vi "Config Write Interface.vi"(8 "error in (no error)":errorcluster, 10 "Device Ref in":T1 format="%.0x", 11 "Refnum in":T2) -> (0 "error out":errorcluster, 2 "Device Ref out":T1 format="%.0x", 3 "Refnum out":T2)   [LabVIEW 2019, in "Modbus Master System Explorer.lvlib"]
uses:
  Modbus Master System Explorer.lvlib
  <vilib>/Utility/config.llb/Config Data RefNum.ctl
  <vilib>/NI VeriStand/Custom Device API/Custom Device Item Ref.ctl
  <vilib>/Utility/config.llb/NI_LVConfig.lvlib
  <vilib>/NI VeriStand/Custom Device API/Custom Device API.lvlib
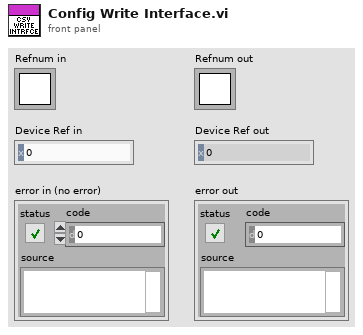
[diagram p1: front panel]
types:
  T1 = typedef "Custom Device API.lvlib/Custom Device Item Ref.ctl" = u64
  T2 = typedef "NI_LVConfig.lvlib/Config Data RefNum.ctl" = refnum<k1>
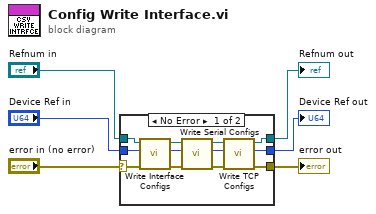
[diagram p0: block diagram]
diagram:
  n1 = case shown="No Error" "error in (no error)" {
    selector: "error in (no error)" -> [w16 w19]
    tunnel: "Refnum in" -> [w18 w21]
    tunnel: "Device Ref in" -> [w17 w20]
    tunnel: [w9 w20] -> w3
    tunnel: [w8 w21] -> w2
    tunnel: [w7 w19] -> w1
    frame No Error {
      n2 = call "Write Interface Configs.vi"("error in (no error)"=w16, "Device Ref in"=w17, "Refnum in"=w18) -> ("error out"=w14:errorcluster, "Item Ref out"=w13:T1, "Refnum out"=w15:T2)  [unwired: 6 in]
      n3 = call "Write Serial Configs.vi"("error in (no error)"=w14, "Item Ref in"=w13, "Refnum in"=w15) -> ("error out"=w11:errorcluster, "Item Ref out"=w12:T1, "Refnum out"=w10:T2)  [unwired: 6 in]
      n4 = call "Write TCP Configs.vi"("error in (no error)"=w11, "Item Ref in"=w12, "Refnum in"=w10) -> ("error out"=w7:errorcluster, "Item Ref out"=w9:T1, "Refnum out"=w8:T2)  [unwired: 6 in]
    }
    frame Error {
    }
  }
  "error out" <- w1
  "Refnum out" <- w2
  "Device Ref out" <- w3
